vi "WeDo.vi"() -> ()   [LabVIEW 2010]
uses:
  SubVIs/LVPresent_Globals.vi
panel:
  in  "WeDo":bool
  # "WeDo"
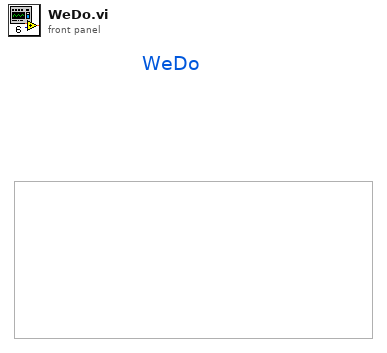
[diagram p1: front panel]
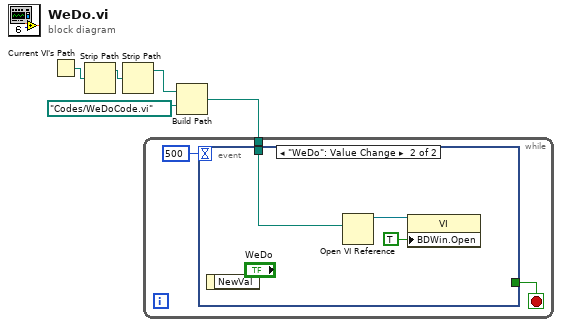
[diagram p0: block diagram]
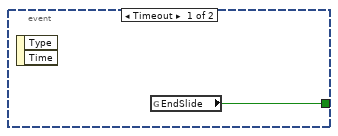
[diagram p2: hidden frame]
diagram:
  n1 = Current VI's Path() -> (path=w5:path)
  n2 = Strip Path(path=w5) -> (stripped path=w4:path)  [unwired: 1 out]
  n3 = Strip Path(path=w4) -> (stripped path=w2:path)  [unwired: 1 out]
  n4 = Build Path(base path=w2, name or relative path=path "Codes/WeDoCode.vi") -> (appended path=w1:path)
  n5 = while {
    tunnel: w1 -> [w6]
    stop <- w8 stop-if-true
    n6 = event shown="[1] \"WeDo\": Value Change" {
      selector: _ -> [_ _]
      dyn-events: _ -> [_ _]
      timeout: 500 -> [_ _]
      tunnel: [w9 _] -> w8
      tunnel: w6 -> [_ w10]
      event Timeout {
        n7 = event-data() -> ()  [unwired: 1 in, 2 out]
        n8 = global read "LVPresent_Globals.vi" "EndSlide"() -> (w9:bool)
      }
      event "WeDo": Value Change {
        n9 = event-data() -> ()  [unwired: 1 in, 1 out]
        n10 = Open VI Reference(vi path=w10) -> (vi reference=w12:refnum<vi>)  [unwired: 5 in, 1 out]
        n11 = property class="VI"(reference=w12, "BDWin.Open"=TRUE ("Block Diagram Window:Open")) -> ()  [unwired: 1 in, 2 out]
      }
    }
  }
